vi "Convert to Waveform.vi"(10 "Data":dbl[][](array[numeric]), 11 "Scan Rate (Hz)":dbl) -> (3 "Waveform":waveform(dbl)[](array[waveform]))   [LabVIEW 2020]
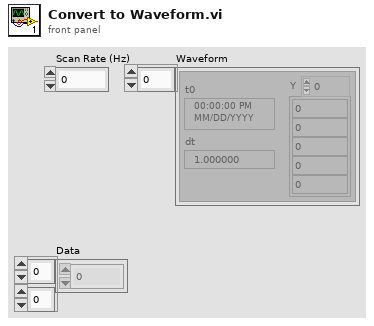
[diagram p1: front panel]
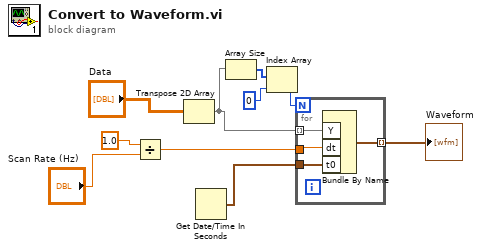
[diagram p0: block diagram]
diagram:
  n1 = Divide(x=1.0, y="Scan Rate (Hz)") -> (x/y=w3:dbl)
  n2 = Transpose 2D Array(2D array="Data") -> (transposed array=w8:dbl[][])
  n3 = Get Date/Time In Seconds() -> (seconds since 1Jan1904=w9:timestamp)
  n4 = Array Size(array=w8) -> (size(s)=w6:i32[])
  n5 = Index Array(array=w6, index=0) -> (element=w5:i32)
  n6 = for {
    N: w5 -> [_]
    tunnel: [w14] -> w10 mode=indexing
    tunnel: w8 -> [w13] mode=indexing
    tunnel: w9 -> [w12]
    tunnel: w3 -> [w11]
    n7 = Bundle By Name("Y"=w13, "dt"=w11, "t0"=w12) -> (w14:waveform(dbl))  [unwired: 1 in]
  }
  "Waveform" <- w10
